vi "Do.vi"(8 "error in (no error)":errorcluster, 9 "Events":refnum<class "Events.lvclass">, 10 "Message Loop Data in":T1, 11 "IInternalRequest in":refnum<class "IHandleSubscribed.lvclass">) -> (0 "error out":errorcluster, 2 "Message Loop Data out":T1, 3 "IInternalRequest out":refnum<class "IHandleSubscribed.lvclass">)   [LabVIEW 2020, in "wamplv.lvlib" / "IHandleSubscribed.lvclass"]
uses:
  IHandleSubscribed.lvclass
  Subscribe/ISubscribe/ISubscribe.lvclass
  WAMP Client/Private/TypeDef/Publish Requests Map.ctl
  wamplv.lvlib
  WAMP Client/Private/TypeDef/Endpoint Data.ctl
  Call/ICallRequest/ICallRequest.lvclass
  WAMP Client/Private/TypeDef/CALL Request Map.ctl
  WAMP Client/Private/TypeDef/SUBSCRIBE Requests Map.ctl
  WAMP Client/Private/TypeDef/Subscriptions Map.ctl
  WAMP Client/Private/TypeDef/Unsubscribe Requests Map.ctl
  WAMP Client/Private/TypeDef/Unregister requests map.ctl
  WAMP Client/Private/TypeDef/Message Loop Data.ctl
  Events/EventsParent/Events.lvclass
  Publish/IPublish/IPublish.lvclass
  Message loop classes/Subscription details/SubscriptionDetailsParent/SubscriptionDetailsParent.lvclass
  Unsubscribe/IUnsubscribe/IUnsubscribe.lvclass
  Register/IRegister/IRegister.lvclass
  Unregister/IUnregister/IUnregister.lvclass
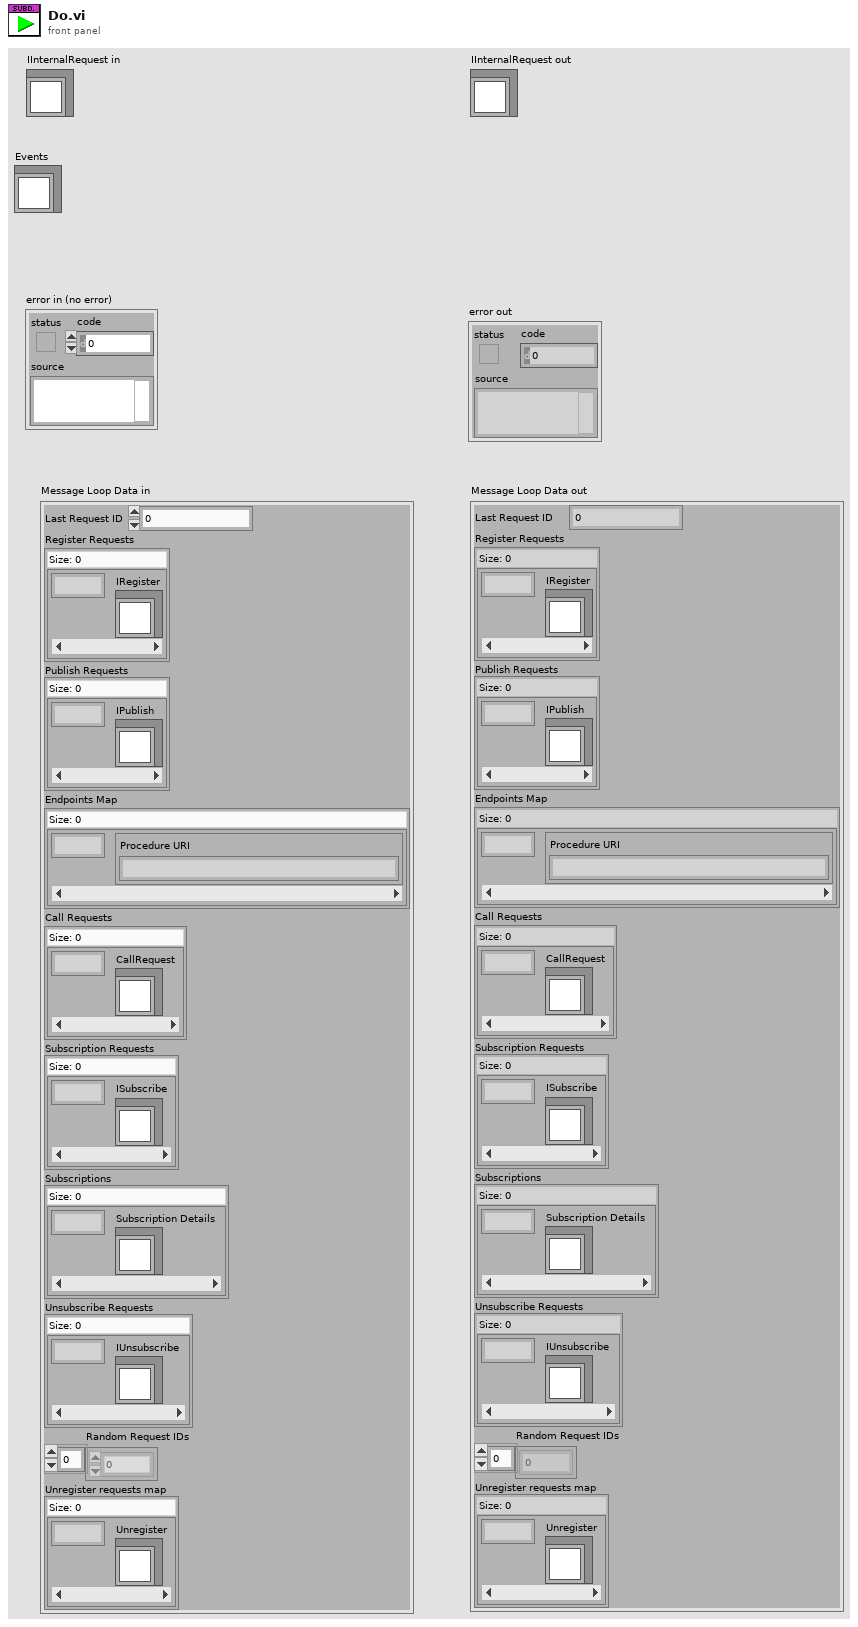
[diagram p1: front panel]
types:
  T1 = typedef "wamplv.lvlib/Message Loop Data.ctl" = cluster{"Last Request ID":u64, "Register Requests":map{u64, refnum<class "IRegister.lvclass">}, "Publish Requests":T2, "Endpoints Map":map{u64, T3}, "Call Requests":T4, "Subscription Requests":T5, "Subscriptions":T6, "Unsubscribe Requests":T7, "Random Request IDs":u64[], "Unregister requests map":T8}
  T2 = typedef "wamplv.lvlib/Publish Requests Map.ctl" = map{u64, refnum<class "IPublish.lvclass">}
  T3 = typedef "wamplv.lvlib/Endpoint Data.ctl" = cluster{"Procedure URI":string}
  T4 = typedef "wamplv.lvlib/CALL Request Map.ctl" = map{u64, refnum<class "ICallRequest.lvclass">}
  T5 = typedef "wamplv.lvlib/SUBSCRIBE Requests Map.ctl" = map{u64, refnum<class "ISubscribe.lvclass">}
  T6 = typedef "wamplv.lvlib/Subscriptions Map.ctl" = map{u64, refnum<class "SubscriptionDetailsParent.lvclass">}
  T7 = typedef "wamplv.lvlib/Unsubscribe Requests Map.ctl" = map{u64, refnum<class "IUnsubscribe.lvclass">}
  T8 = typedef "wamplv.lvlib/Unregister requests map.ctl" = map{u64, refnum<class "IUnregister.lvclass">}
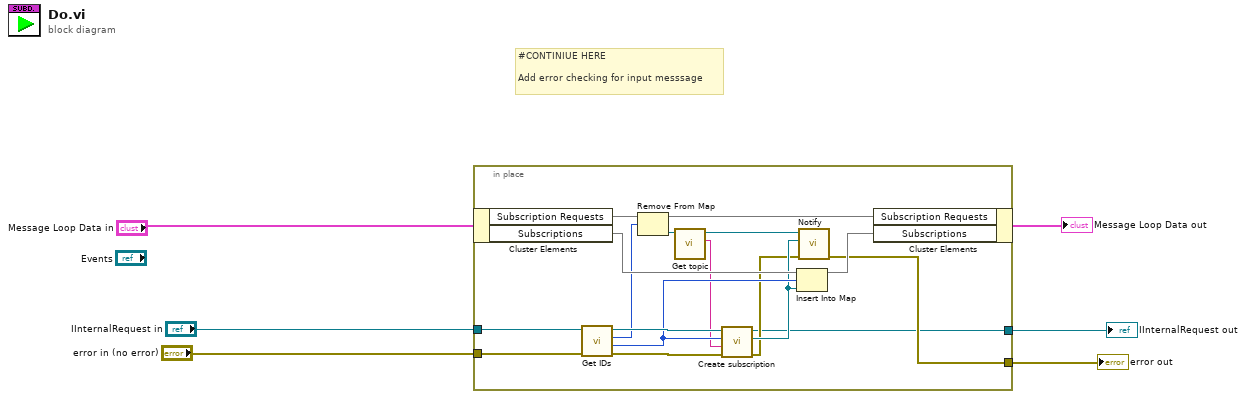
[diagram p0: block diagram]
diagram:
  # "#CONTINIUE HERE\n\nAdd error checking for input messsage"
  n1 = in-place {
    in-place-border: "IInternalRequest in" -> [w18]
    in-place-border: "error in (no error)" -> [w9]
    in-place-border: [w8] -> w2
    in-place-border: [w7] -> w1
    n2 = in-place-cluster #1("Message Loop Data in") -> ("Subscription Requests"=w22:T5, "Subscriptions"=w21:T6)
    n3 = call-dynamic "Get IDs.vi"("error in (no error)"=w9, "IHandleSubscribed in"=w18) -> ("error out"=w19:errorcluster, "Subscription ID"=w16:u64, "Subscription Request ID"=w17:u64, "IHandleSubscribed out"=w20:refnum<class "IHandleSubscribed.lvclass">)  [unwired: 6 in]
    n4 = Remove From Map(10:w17, 11:w22) -> (1:w15:refnum<class "ISubscribe.lvclass">, 3:w23:T5)  [unwired: 1 out]
    n5 = call-dynamic "Get topic.vi"("ISubscribe in"=w15) -> ("Topic"=w14:string, "ISubscribe out"=w12:refnum<class "ISubscribe.lvclass">)  [unwired: 9 in]
    n6 = call-dynamic "Create subscription.vi"("error in (no error)"=w19, "Topic"=w14, "Subscription ID"=w16, "IHandleSubscribed in"=w20) -> ("error out"=w10:errorcluster, "SubscriptionDetailsParent"=w11:refnum<class "SubscriptionDetailsParent.lvclass">, "IHandleSubscribed out"=w7:refnum<class "IHandleSubscribed.lvclass">)  [unwired: 5 in]
    n7 = Insert Into Map(map in=w21, key=w16, value=w11) -> (map out=w13:T6)  [unwired: 2 out]
    n8 = call-dynamic "Notify.vi"("error in (no error)"=w10, "SubscriptionDetailsParent"=w11, "ISubscribe in"=w12) -> ("error out"=w8:errorcluster)  [unwired: 7 in, 1 out]
    n9 = in-place-cluster #1("Subscription Requests"=w23, "Subscriptions"=w13) -> (→"Message Loop Data out":T1)
  }
  "error out" <- w2
  "IInternalRequest out" <- w1
